vi "LCR_SendAll.vi"(8 "error in (no error)":errorcluster, 10 "Configuration Cluster":T1={"General"={"Config.ini"=path "", "Default Logging Path"=path ""}, "Hardware"={"AHC VISA COM"="", "Measure Rate (1/s)"=0, "Global T VAR"="", "Global B VAR"=""}, "Operation"={"Operation Mode"=enum."Idle-Off", "Status"="", "NewLog?"=FALSE}}, 11 "VISA resource name":refnum<visa-resource-name>) -> (0 "error out":errorcluster, 2 "Configuration Cluster Out":T1={"General"={"Config.ini"=path "", "Default Logging Path"=path ""}, "Hardware"={"AHC VISA COM"="", "Measure Rate (1/s)"=0, "Global T VAR"="", "Global B VAR"=""}, "Operation"={"Operation Mode"=enum."Idle-Off", "Status"="", "NewLog?"=FALSE}}, 3 "VISA resource name out":refnum<visa-resource-name>)   [LabVIEW 2021]
uses:
  <instrlib>/Hameg HM8118/Hameg HM8118.lvlib
  Config_Cluster.ctl
  Mode_Enum.ctl
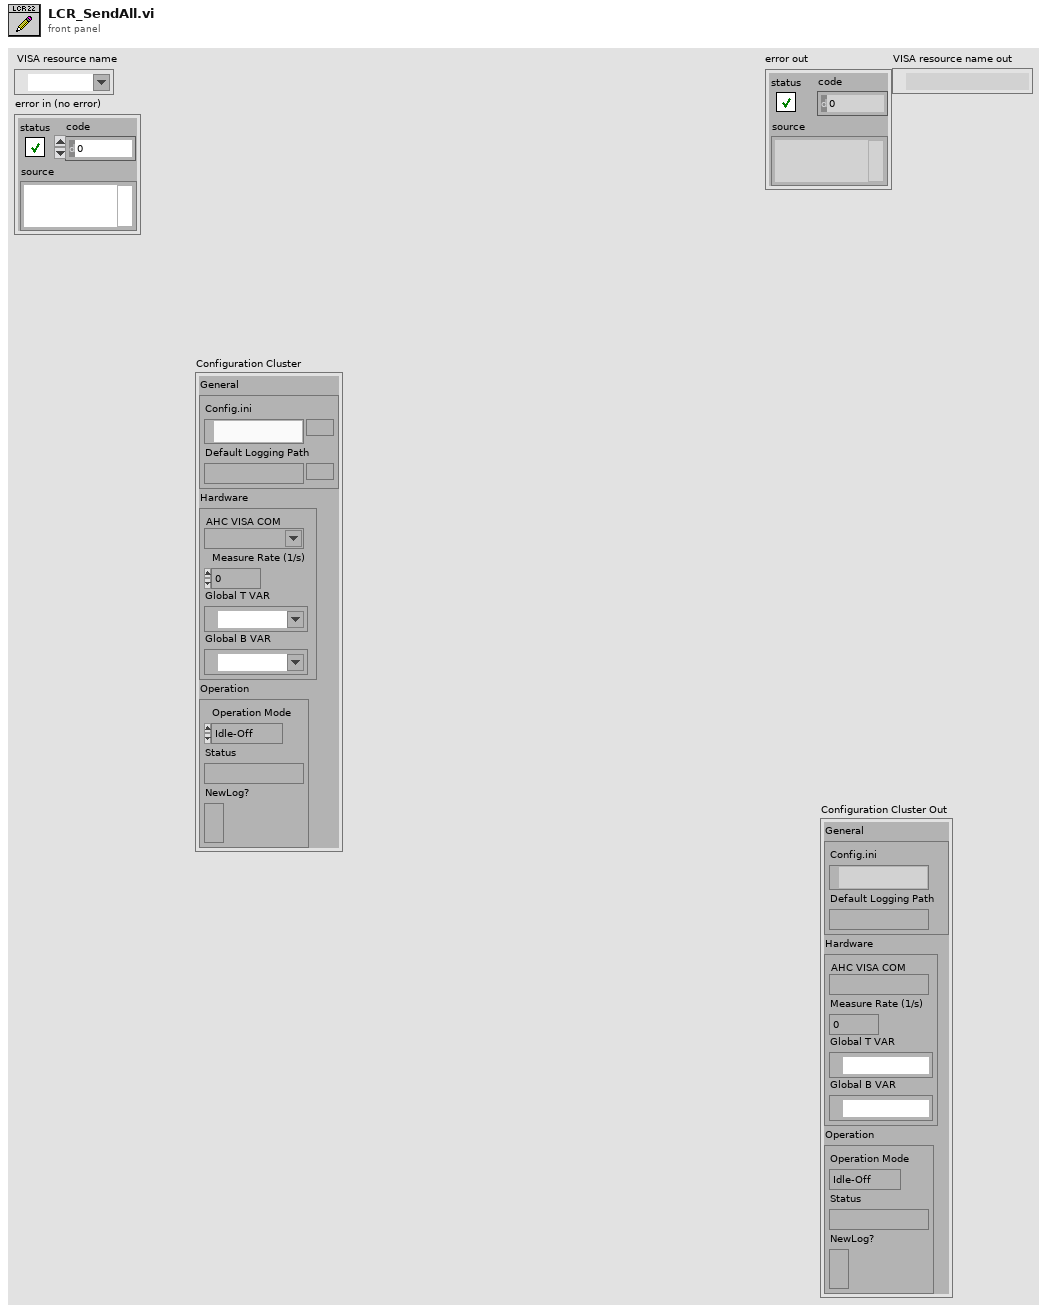
[diagram p1: front panel]
types:
  T1 = typedef "Config_Cluster.ctl" = cluster{"General":cluster{"Config.ini":path, "Default Logging Path":path}, "Hardware":cluster{"AHC VISA COM":refnum<visa-resource-name>, "Measure Rate (1/s)":i32, "Global T VAR":refnum<k21>, "Global B VAR":refnum<k21>}, "Operation":cluster{"Operation Mode":T2, "Status":string, "NewLog?":bool}}
  T2 = typedef "Mode_Enum.ctl" = enum16{"Logging", "Idle-Off", "Idle"}
  T3 = cluster{"Bias Profile":cluster{" Bias Source (OFF)":u8, " Bias Type (Voltage)":u8, "Bias Level (0)":dbl}, "Measurement Profile":cluster{"Operation Mode (0: Auto)":u16, "Circuit Type (2: Auto)":u16, "Manual Range (1:Range 1 and 25 Ohms)":u8, "Auto Range (T: Enable)":bool}, "Signal Profile":cluster{"Frequency (1kHz)":dbl, "Measuring Voltage (1V)":dbl}, "Integration Profile":cluster{"Averaging (0: Off)":u16, "Averaging Number (2)":i32, "Time (100ms)":i32, "Rate (0: Fast)":u16}, "Trigger Profile":cluster{"Trigger Mode (0: Continuous)":u16}}
  T4 = cluster{" Bias Source (OFF)":u8, " Bias Type (Voltage)":u8, "Bias Level (0)":dbl}
  T5 = cluster{"Operation Mode (0: Auto)":u16, "Circuit Type (2: Auto)":u16, "Manual Range (1:Range 1 and 25 Ohms)":u8, "Auto Range (T: Enable)":bool}
  T6 = cluster{"Frequency (1kHz)":dbl, "Measuring Voltage (1V)":dbl}
  T7 = cluster{"Averaging (0: Off)":u16, "Averaging Number (2)":i32, "Time (100ms)":i32, "Rate (0: Fast)":u16}
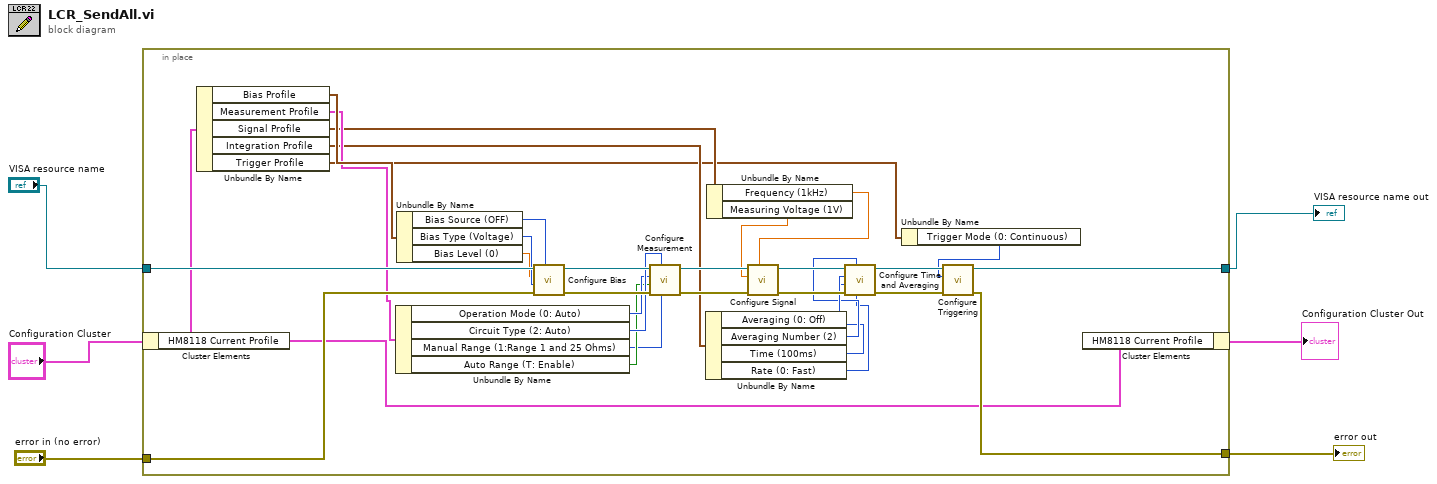
[diagram p0: block diagram]
diagram:
  n1 = in-place {
    in-place-border: "VISA resource name" -> [w38]
    in-place-border: "error in (no error)" -> [w29]
    in-place-border: [w28] -> w4
    in-place-border: [w27] -> w3
    n2 = in-place-cluster #1("Configuration Cluster") -> ("HM8118 Current Profile"=w12:T3)
    n3 = Unbundle By Name(w12) -> ("Bias Profile"=w11:T4, "Measurement Profile"=w10:T5, "Signal Profile"=w9:T6, "Integration Profile"=w8:T7, "Trigger Profile"=w7:cluster{"Trigger Mode (0: Continuous)":u16})
    n4 = Unbundle By Name(w10) -> ("Operation Mode (0: Auto)"=w22:u16, "Circuit Type (2: Auto)"=w23:u16, "Manual Range (1:Range 1 and 25 Ohms)"=w20:u8, "Auto Range (T: Enable)"=w21:bool)
    n5 = Unbundle By Name(w11) -> ("Bias Source (OFF)"=w26:u8, "Bias Type (Voltage)"=w25:u8, "Bias Level (0)"=w24:dbl)
    n6 = call <instrlib>:"Configure Bias.vi"("Bias Source (OFF)"=w26, "error in (no error)"=w29, "Bias Type (Voltage)"=w25, "Bias Level (0)"=w24, "VISA resource name"=w38) -> ("error out"=w33:errorcluster, "VISA resource name out"=w37:refnum<visa-resource-name>)  [unwired: 5 in]
    n7 = call <instrlib>:"Configure Measurement.vi"("Manual Range (1:Range 1 and 25 Ohms)"=w20, "Circuit Type (2: Auto)"=w23, "error in (no error)"=w33, "Auto Range (T: Enable)"=w21, "Operation Mode (0: Auto)"=w22, "VISA resource name"=w37) -> ("error out"=w32:errorcluster, "VISA resource name out"=w36:refnum<visa-resource-name>)  [unwired: 4 in]
    n8 = Unbundle By Name(w8) -> ("Averaging (0: Off)"=w17:u16, "Averaging Number (2)"=w16:i32, "Time (100ms)"=w15:i32, "Rate (0: Fast)"=w14:u16)
    n9 = Unbundle By Name(w9) -> ("Frequency (1kHz)"=w19:dbl, "Measuring Voltage (1V)"=w18:dbl)
    n10 = call <instrlib>:"Configure Signal.vi"("Frequency (1kHz)"=w19, "error in (no error)"=w32, "Measuring Voltage (1V)"=w18, "VISA resource name"=w36) -> ("error out"=w31:errorcluster, "VISA resource name out"=w35:refnum<visa-resource-name>)  [unwired: 6 in]
    n11 = call <instrlib>:"Configure Time and Averaging.vi"("Rate (0: Fast)"=w14, "Averaging Number (2)"=w16, "error in (no error)"=w31, "Time (100ms)"=w15, "Averaging (0: Off)"=w17, "VISA resource name"=w35) -> ("error out"=w30:errorcluster, "VISA resource name out"=w34:refnum<visa-resource-name>)  [unwired: 4 in]
    n12 = Unbundle By Name(w7) -> ("Trigger Mode (0: Continuous)"=w13:u16)
    n13 = call <instrlib>:"Configure Triggering.vi"("error in (no error)"=w30, "Trigger Mode (0: Continuous)"=w13, "VISA resource name"=w34) -> ("error out"=w28:errorcluster, "VISA resource name out"=w27:refnum<visa-resource-name>)  [unwired: 7 in]
    n14 = in-place-cluster #1("HM8118 Current Profile"=w12) -> (→"Configuration Cluster Out":T1)
  }
  "error out" <- w4
  "VISA resource name out" <- w3
